vi "WaitForCommand.vi"(8 "error in (no error)":errorcluster, 11 "ServiceManager-Comms in":refnum<class "ServiceManager-Comms.lvclass">) -> (0 "error out":errorcluster, 3 "ServiceManager-Comms out":refnum<class "ServiceManager-Comms.lvclass">)   [LabVIEW 2020, in "ServiceManager.lvlib" / "ServiceManager-Comms.lvclass"]
uses:
  ServiceManager-Comms.lvclass
  C:/Program Files (x86)/National Instruments/LabVIEW 2020/vi.lib/ActorFramework/Actor/Actor.lvclass
  ServiceManager-Comms Messages/WaitForCommand Msg/WaitForCommand Msg.lvclass
  C:/Program Files (x86)/National Instruments/LabVIEW 2020/vi.lib/ActorFramework/Message/Message.lvclass
  ServiceManager/DownstreamMsg/DownStreamMsgHandler.lvclass
  <vilib>/ActorFramework/Actor/Actor.lvclass
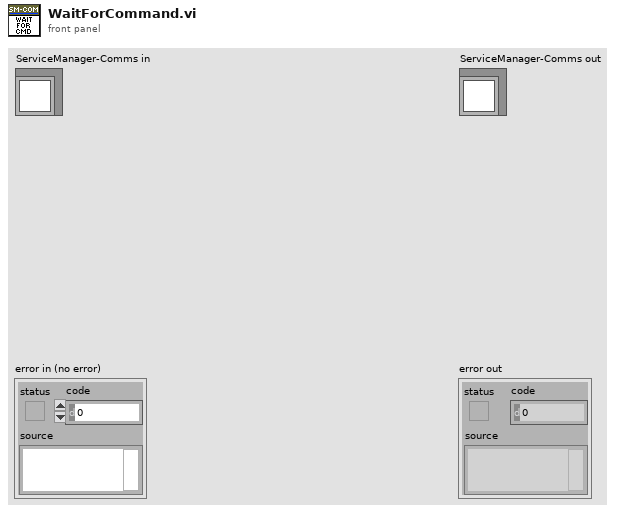
[diagram p1: front panel]
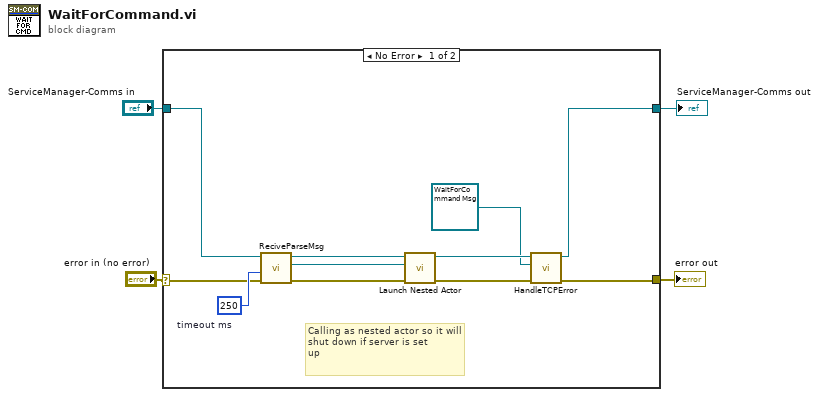
[diagram p0: block diagram]
diagram:
  n1 = case shown="No Error" "error in (no error)" {
    selector: "error in (no error)" -> [w14 w17]
    tunnel: [w5 w17] -> w3
    tunnel: [w6 w16] -> w1
    tunnel: "ServiceManager-Comms in" -> [w10 w16]
    frame No Error {
      w15 = 250  # timeout ms
      # "Calling as nested actor so it will shut down if server is set \nup"
      n2 = call-dynamic "ReciveParseMsg.vi"("error in (no error)"=w14, "timeout ms (25000)"=w15, "ServiceManager-Comms in"=w10) -> ("error out"=w11:errorcluster, "DownStreamMsgHandler"=w13:refnum<class "DownStreamMsgHandler.lvclass">, "ServiceManager-Comms out"=w12:refnum<class "ServiceManager-Comms.lvclass">)  [unwired: 6 in]
      n3 = call <vilib>:"Launch Nested Actor.vi"("error in (no error)"=w11, "Nested Actor"=w13, "Caller Actor in"=w12) -> ("error out"=w8:errorcluster, "Caller Actor out"=w9:refnum<class "ServiceManager-Comms.lvclass">)  [unwired: 6 in, 1 out]
      n4 = call "HandleTCPError.vi"("error in (no error)"=w8, "NoErrorMessage"=refnum<class "WaitForCommand Msg.lvclass"> refnum ("ServiceManager.lvlib:WaitForCommand Msg.lvclass"), "ServiceManager-Comms in"=w9) -> ("error out"=w5:errorcluster, "ServiceManager-Comms out"=w6:refnum<class "ServiceManager-Comms.lvclass">)  [unwired: 7 in]
    }
    frame Error {
    }
  }
  "error out" <- w3
  "ServiceManager-Comms out" <- w1
